vi "Y stage safety.vi"(7 "new position":dbl format="%#_13g", 8 "Error In":errorcluster, 10 "Table Stages":T1={"X Stage"={"Position"=0.0, "Is.Enabled?"=FALSE, "Is.Connected?"=FALSE, "Device SN"="45876539", "AccelerationMaximum"=0.0, "VelocityMaximum"=0.0, "Acceleration"=0.0, "Velocity"=0.0, "waitTimeout (ms)"=0, "Model"=enum."None", "Is.Homed?"=FALSE, "MOVE"=FALSE}, "Y Stage"={"Position"=0.0, "Is.Enabled?"=FALSE, "Is.Connected?"=FALSE, "Device SN"="45876539", "AccelerationMaximum"=0.0, "VelocityMaximum"=0.0, "Acceleration"=0.0, "Velocity"=0.0, "waitTimeout (ms)"=0, "Model"=enum."None", "Is.Homed?"=FALSE, "MOVE"=FALSE}, "Z Stage"={"Position"=0.0, "Is.Enabled?"=FALSE, "Is.Connected?"=FALSE, "Device SN"="45876539", "AccelerationMaximum"=0.0, "VelocityMaximum"=0.0, "Acceleration"=0.0, "Velocity"=0.0, "waitTimeout (ms)"=0, "Model"=enum."None", "Is.Homed?"=FALSE, "MOVE"=FALSE}, "Attenuator"={"Position"=0.0, "Is.Enabled?"=FALSE, "Is.Connected?"=FALSE, "Device SN"="45876539", "AccelerationMaximum"=0.0, "VelocityMaximum"=0.0, "Acceleration"=0.0, "Velocity"=0.0, "waitTimeout (ms)"=0, "Model"=enum."None", "Is.Homed?"=FALSE, "MOVE"=FALSE}}) -> (0 "Error Out":errorcluster, 1 "crash?":bool, 2 "Table Stages [out]":T1={"X Stage"={"Position"=0.0, "Is.Enabled?"=FALSE, "Is.Connected?"=FALSE, "Device SN"="45876539", "AccelerationMaximum"=0.0, "VelocityMaximum"=0.0, "Acceleration"=0.0, "Velocity"=0.0, "waitTimeout (ms)"=0, "Model"=enum."None", "Is.Homed?"=FALSE, "MOVE"=FALSE}, "Y Stage"={"Position"=0.0, "Is.Enabled?"=FALSE, "Is.Connected?"=FALSE, "Device SN"="45876539", "AccelerationMaximum"=0.0, "VelocityMaximum"=0.0, "Acceleration"=0.0, "Velocity"=0.0, "waitTimeout (ms)"=0, "Model"=enum."None", "Is.Homed?"=FALSE, "MOVE"=FALSE}, "Z Stage"={"Position"=0.0, "Is.Enabled?"=FALSE, "Is.Connected?"=FALSE, "Device SN"="45876539", "AccelerationMaximum"=0.0, "VelocityMaximum"=0.0, "Acceleration"=0.0, "Velocity"=0.0, "waitTimeout (ms)"=0, "Model"=enum."None", "Is.Homed?"=FALSE, "MOVE"=FALSE}, "Attenuator"={"Position"=0.0, "Is.Enabled?"=FALSE, "Is.Connected?"=FALSE, "Device SN"="45876539", "AccelerationMaximum"=0.0, "VelocityMaximum"=0.0, "Acceleration"=0.0, "Velocity"=0.0, "waitTimeout (ms)"=0, "Model"=enum."None", "Is.Homed?"=FALSE, "MOVE"=FALSE}})   [LabVIEW 2018]
uses:
  Controls/Translation Stage Parameters.ctl
  Hardware Mfg/Thorlabs Translation Stages/Controls/Translation Stage Cluster.ctl
  Controls/Translation Stage Types.ctl
  Controls/Set Get Controls.ctl
  Hardware Mfg/Thorlabs Translation Stages/Controls/Motion Translation Module Control2.ctl
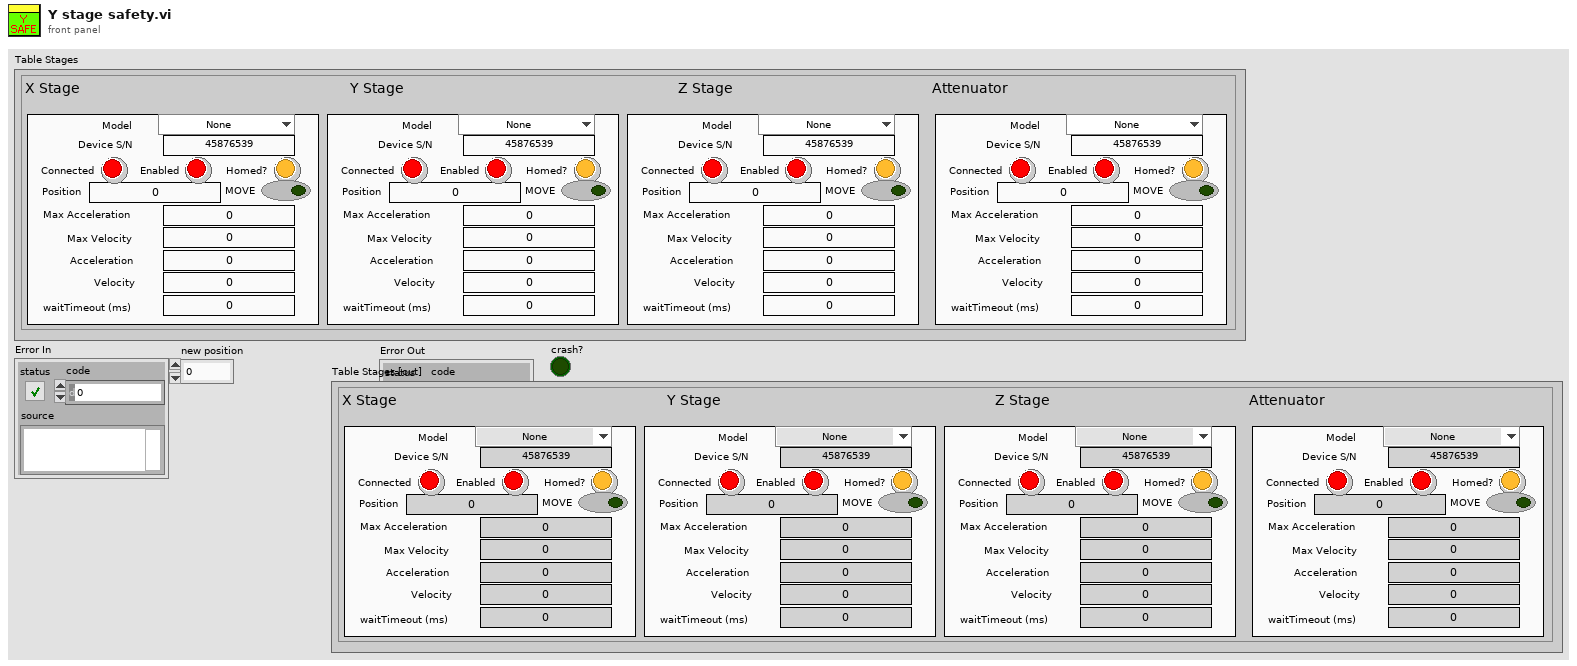
[diagram p1: front panel]
types:
  T1 = typedef "Translation Stage Parameters.ctl" = cluster{"X Stage":T2, "Y Stage":T2, "Z Stage":T2, "Attenuator":T2}
  T2 = typedef "Translation Stage Cluster.ctl" = cluster{"Position":dbl, "Is.Enabled?":bool, "Is.Connected?":bool, "Device SN":string, "AccelerationMaximum":dbl, "VelocityMaximum":dbl, "Acceleration":dbl, "Velocity":dbl, "waitTimeout (ms)":i32, "Model":T3, "Is.Homed?":bool, "MOVE":bool}
  T3 = typedef "Translation Stage Types.ctl" = enum16{"None", "Thorlabs LTS", "Thorlabs MLJ"}
  T4 = typedef "Motion Translation Module Control2.ctl" = enum16{"Init", "Home", "Status", "Velocity/Accel", "Position", "Jog", "Stop", "Uninit", "Enable", "Disable"}
  T5 = typedef "Set Get Controls.ctl" = enum16{"Set", "Get"}
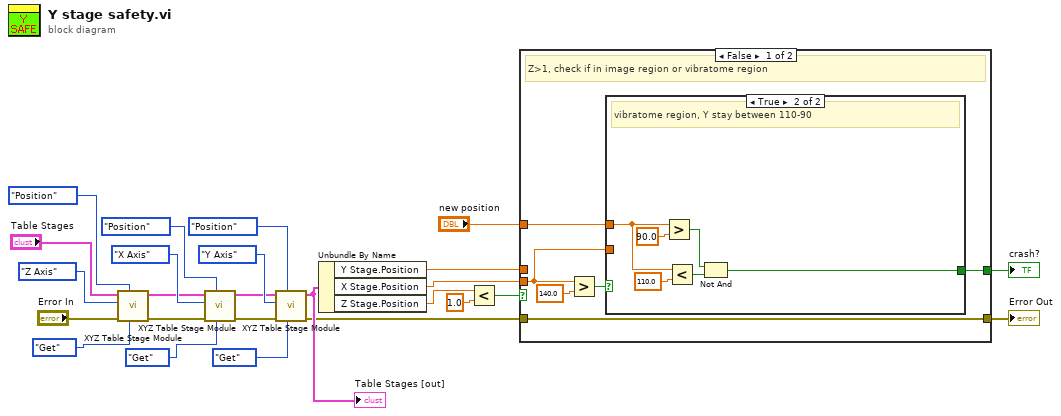
[diagram p0: block diagram]
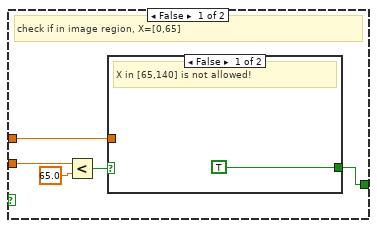
[diagram p2: hidden frame]
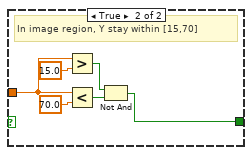
[diagram p3: hidden frame]
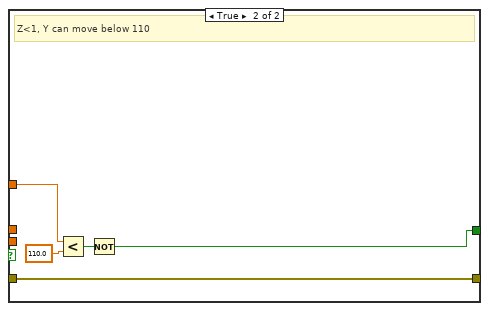
[diagram p4: hidden frame]
diagram:
  n1 = call "XYZ Table Stage Module.vi"("Set/Get"=Set_Get_Controls."Get", "Action"=Motion_Translation_Module_Control2."Position", "Error In"="Error In", "Axis"=enum16{"X Axis", "Y Axis", "Z Axis"}."Z Axis", "Table Stages"="Table Stages") -> ("Error Out"=w18:errorcluster, "Table Stages [out]"=w2:T1)  [unwired: 5 in]
  n2 = call "XYZ Table Stage Module.vi"("Set/Get"=Set_Get_Controls."Get", "Action"=Motion_Translation_Module_Control2."Position", "Error In"=w18, "Axis"=enum16{"X Axis", "Y Axis", "Z Axis"}."X Axis", "Table Stages"=w2) -> ("Error Out"=w14:errorcluster, "Table Stages [out]"=w1:T1)  [unwired: 5 in]
  n3 = call "XYZ Table Stage Module.vi"("Set/Get"=Set_Get_Controls."Get", "Action"=Motion_Translation_Module_Control2."Position", "Error In"=w14, "Axis"=enum16{"X Axis", "Y Axis", "Z Axis"}."Y Axis", "Table Stages"=w1) -> ("Error Out"=w6:errorcluster, "Table Stages [out]"=w13:T1)  [unwired: 5 in]
  "Table Stages [out]" <- w13
  n4 = Unbundle By Name(w13) -> ("Y Stage.Position"=w9:dbl, "X Stage.Position"=w4:dbl, "Z Stage.Position"=w3:dbl)
  n5 = Less?(x=w3, y=1.0) -> (x < y?=w11:bool)
  n6 = case shown="False" w11 {
    tunnel: "new position" -> [w28 w50]
    tunnel: w9 -> [_ _]
    tunnel: [w27 w52] -> w8
    tunnel: w4 -> [w26 _]
    tunnel: w6 -> [w31 w51]
    tunnel: [w31 w51] -> w5
    frame False {
      # "Z>1, check if in image region or vibratome region"
      n7 = Greater?(x=w26, y=140.0) -> (0:w29:bool)
      n8 = case shown="True" w29 {
        tunnel: w28 -> [w33 w48]
        tunnel: [w32 w44] -> w27
        tunnel: w26 -> [w36 _]
        frame False {
          # "check if in image region, X=[0,65]"
          n9 = Less?(x=w36, y=65.0) -> (x < y?=w34:bool)
          n10 = case shown="False" w34 {
            tunnel: w33 -> [_ w39]
            tunnel: [TRUE w38] -> w32
            frame False {
              # "X in [65,140] is not allowed!"
            }
            frame True {
              # "In image region, Y stay within [15,70]"
              n11 = Greater?(x=w39, y=15.0) -> (0:w41:bool)
              n12 = Less?(x=w39, y=70.0) -> (x < y?=w40:bool)
              n13 = Not And(1:w40, 2:w41) -> (0:w38:bool)
            }
          }
        }
        frame True {
          # "vibratome region, Y stay between 110-90"
          n14 = Greater?(x=w48, y=90.0) -> (0:w46:bool)
          n15 = Less?(x=w48, y=110.0) -> (x < y?=w45:bool)
          n16 = Not And(1:w45, 2:w46) -> (0:w44:bool)
        }
      }
    }
    frame True {
      # "Z<1, Y can move below 110"
      n17 = Less?(x=w50, y=110.0) -> (x < y?=w53:bool)
      n18 = Not(x=w53) -> (.not. x?=w52:bool)
    }
  }
  "crash?" <- w8
  "Error Out" <- w5
